vi "ke37xx DMM Configuration Catalog.vi"(0 "VISA Resource Name":refnum<visa-resource-name>, 11 "error in (no error)":errorcluster, 12 "Bytes To Read (1024)":u32=1024) -> (4 "VISA Resource Name Out":refnum<visa-resource-name>, 8 "Configuration Names":string[](array[string]), 15 "error out":errorcluster)   [LabVIEW 2009, in "Keithley 3700 Series.lvlib"]
doc: "This VI queries the system for all of the currently defined DMM configurations."
uses:
  <instrlib>/Keithley 3706/Keithley 3700 Series.lvlib
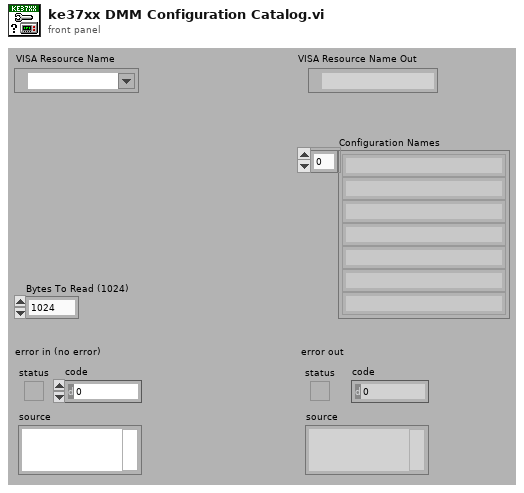
[diagram p1: front panel]
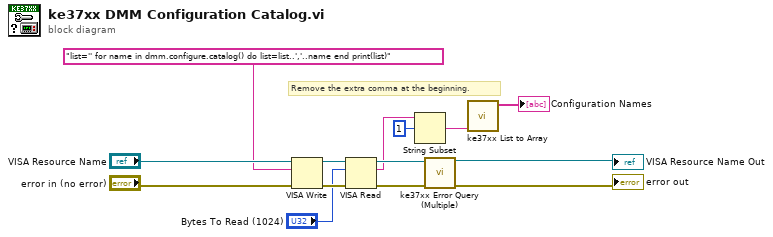
[diagram p0: block diagram]
diagram:
  # "Remove the extra comma at the beginning."
  n1 = VISA Write(VISA resource name="VISA Resource Name", write buffer="list='' for name in dmm.configure.catalog() do list=list..','..name end print(list)", error in (no error)="error in (no error)") -> (VISA resource name out=w10:refnum<visa-resource-name>, error out=w8:errorcluster)  [unwired: 1 out]
  n2 = VISA Read(VISA resource name=w10, byte count="Bytes To Read (1024)", error in (no error)=w8) -> (VISA resource name out=w9:refnum<visa-resource-name>, read buffer=w3:string, error out=w7:errorcluster)  [unwired: 1 out]
  n3 = String Subset(string=w3, offset (0)=1) -> (substring=w1:string)  [unwired: 1 out]
  n4 = call <instrlib>:"ke37xx Error Query (Multiple).vi"("VISA resource name"=w9, "error in (no error)"=w7) -> ("VISA resource name out"=→"VISA Resource Name Out":refnum<visa-resource-name>, "error out"=→"error out":errorcluster)  [unwired: 12 out]
  n5 = call <instrlib>:"ke37xx List to Array.vi"("List"=w1) -> ("Output String Array"=→"Configuration Names":string[])  [unwired: 1 in, 5 out]
